vi "To Nested Variant.vi"(11 "variant in":variant) -> (3 "variant out":variant)   [LabVIEW 2015, in "LV String Utils v1.lvlib"]
doc: "Replaces two occurances of 'To Variant' function."
uses:
  LV String Utils v1.lvlib
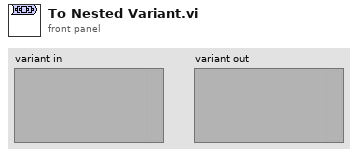
[diagram p1: front panel]
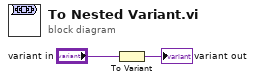
[diagram p0: block diagram]
diagram:
  n1 = To Variant(anything="variant in") -> (Variant=→"variant out":variant)
